vi "4 Sigma Filter.vi"(11 "Input Data":dbl[](array[numeric])) -> (2 "mean":dbl, 3 "Histogram Graph":T1)   [LabVIEW 2016]
uses:
  <vilib>/Analysis/baseanly.llb/Mean (DBL).vi
  <vilib>/Analysis/baseanly.llb/Unimode.vi
  <vilib>/Analysis/NI_AALBase.lvlib
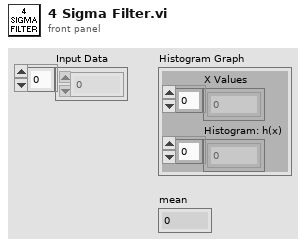
[diagram p1: front panel]
types:
  T1 = cluster{"X Values":dbl[], "Histogram: h(x)":i32[]}
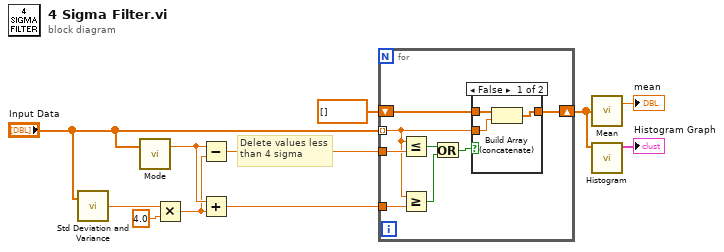
[diagram p0: block diagram]
diagram:
  # "Delete values less\nthan 4 sigma"
  n1 = call <vilib>:"Std Deviation and Variance.vi"("X"="Input Data") -> ("standard deviation"=w5:dbl)  [unwired: 1 in, 2 out]
  n2 = call-poly <vilib>:"Mode.vi"("X"="Input Data") -> ("mode"=w3:dbl)  [unwired: 1 in, 1 out]
  n3 = Multiply(x=w5, y=4.0) -> (x*y=w2:dbl)
  n4 = Subtract(x=w3, y=w2) -> (x-y=w9:dbl)
  n5 = Add(x=w3, y=w2) -> (x+y=w1:dbl)
  n6 = for {
    tunnel: "Input Data" -> [w15] mode=indexing
    shift-right: [w18] -> w10
    shift-left: dbl[] [] -> [w19]
    tunnel: w9 -> [w17]
    tunnel: w1 -> [w16]
    n7 = Less Or Equal?(x=w15, y=w17) -> (x <= y?=w13:bool)
    n8 = Greater Or Equal?(x=w15, y=w16) -> (x >= y?=w14:bool)
    n9 = Or(x=w13, y=w14) -> (x .or. y?=w12:bool)
    n10 = case shown="False" w12 {
      tunnel: w19 -> [w22 w23]
      tunnel: [w21 w23] -> w18
      tunnel: w15 -> [w20 _]
      frame False {
        n11 = Build Array (concatenate)(w22, w20) -> (w21:dbl[])
      }
      frame True {
      }
    }
  }
  n12 = call-poly <vilib>:"Mean.vi"("X"=w10) -> ("mean"=→"mean":dbl)  [unwired: 1 out]
  n13 = call <vilib>:"Histogram.vi"("X"=w10) -> ("Histogram Graph"=→"Histogram Graph":T1)  [unwired: 7 in, 3 out]
